vi "IO@ClrPort__Parameter.vi"(1 "ParamterIn":string) -> (0 "ParamterOut":string)   [LabVIEW 2019]
panel:
  in  "Delay":string(combo)
  in  "PortSelect":string(combo)
  in  "Confirm":bool
  # "IO@SetPort/ClrPort $IOName(,$Delay)"
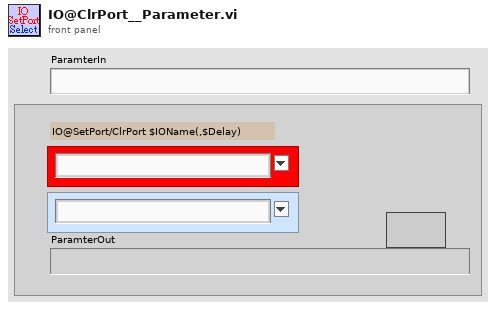
[diagram p1: front panel]
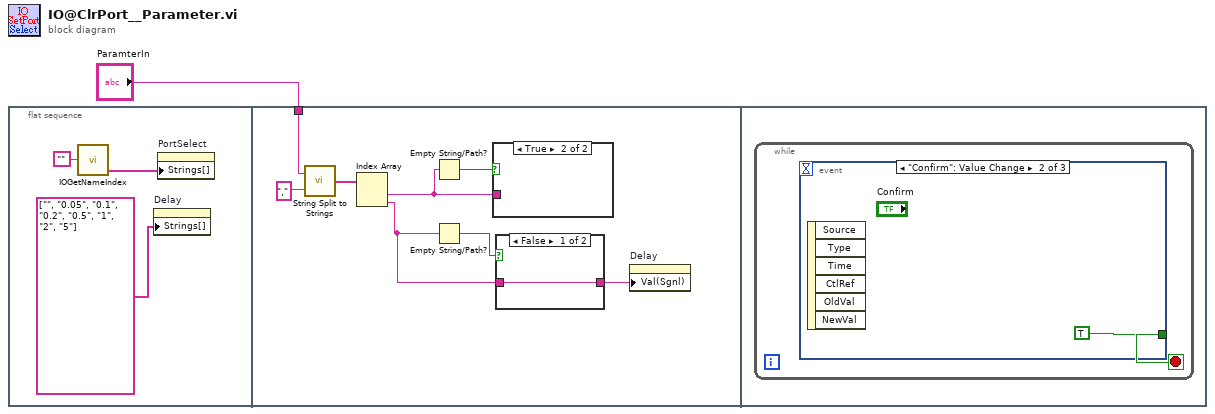
[diagram p0: block diagram]
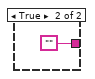
[diagram p2: hidden frame]
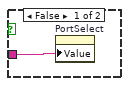
[diagram p3: hidden frame]
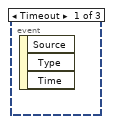
[diagram p4: hidden frame]
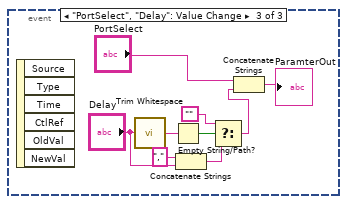
[diagram p5: hidden frame]
diagram:
  n1 = flat-sequence {
    tunnel: "ParamterIn" -> [w10]
    frame #0 {
      n2 = call "IOGetNameIndex.vi"("PortName"="") -> ("PortNameList Out"=w3:string[])  [unwired: 3 in, 1 out]
      n3 = property on="Delay" class="CmbBox"("Strings[]"=string[] ["", "0.05", "0.1", "0.2", "0.5", "1", "2", "5"] ("Strings []")) -> ()  [unwired: 2 in, 2 out]
      n4 = property on="PortSelect" class="CmbBox"("Strings[]"=w3) -> ()  [unwired: 2 in, 2 out]
    }
    frame #1 {
      n5 = call "String Split to Strings.vi"("search string/char (-)"=",", "String"=w10) -> ("Array"=w11:string[])
      n6 = Index Array(array=w11) -> (element #1=w8:string, element #2=w5:string)  [unwired: 2 in]
      n7 = Empty String/Path?(string/path=w8) -> (empty?=w9:bool)
      n8 = Empty String/Path?(string/path=w5) -> (empty?=w7:bool)
      n9 = case shown="True" w9 {
        tunnel: w8 -> [w15 _]
        frame False {
          n10 = property on="PortSelect" class="CmbBox"("Value"=w15) -> ()  [unwired: 2 in, 2 out]
        }
        frame True {
        }
      }
      n11 = case shown="False" w7 {
        tunnel: [w13 ""] -> w6
        tunnel: w5 -> [w13 _]
        frame False {
        }
        frame True {
        }
      }
      n12 = property on="Delay" class="CmbBox"("Val(Sgnl)"=w6) -> ()  [unwired: 2 in, 2 out]
    }
    frame #2 {
      n13 = while {
        stop <- w16 stop-if-true
        n14 = event shown="[1] \"Confirm\": Value Change" {
          selector: _ -> [_ _ _]
          dyn-events: _ -> [_ _ _]
          timeout: _ -> [_ _ _]
          tunnel: [_ TRUE _] -> w16
          event Timeout {
            n15 = event-data() -> ()  [unwired: 1 in, 3 out]
          }
          event "Confirm": Value Change {
            n16 = event-data() -> ()  [unwired: 1 in, 6 out]
          }
          event "PortSelect", "Delay": Value Change {
            n17 = event-data() -> ()  [unwired: 1 in, 6 out]
            n18 = call <vilib>:"Trim Whitespace.vi"("string"="Delay") -> ("trimmed string"=w24:string)  [unwired: 1 in]
            n19 = Empty String/Path?(string/path=w24) -> (empty?=w23:bool)
            n20 = Concatenate Strings("," ("string"), "Delay") -> (w21:string)
            n21 = Select(t="", s=w23, f=w21) -> (s? t:f=w18:string)
            n22 = Concatenate Strings("PortSelect", w18) -> (→"ParamterOut":string)
          }
        }
      }
    }
  }
